vi "Basic.vi"() -> ()   [LabVIEW 2016, in "DronaTest.lvlib" / "test_ValueSignal.lvlib"]
uses:
  test_ValueSignal.lvlib
  main/apis/Setup/GetVI/GetVIByPath.vi
  main/apis/Stimulus/ValueSignal/ValueSignalByPathString.vi
  main/apis/Assert/AssertControlValue/Equal.vi
  main/apis/Assert/AssertControlValue/True.vi
  main/Drona.lvlib
  main/apis/Setup/GetVI/GetVI.lvlib
  <vilib>/addons/_JKI Toolkits/Caraya/classes/Test/Test.lvclass
  main/apis/Stimulus/ValueSignal/ValueSignal.lvlib
  main/apis/Assert/AssertControlValue/AssertControlValue.lvlib
panel:
  out "error out":errorcluster
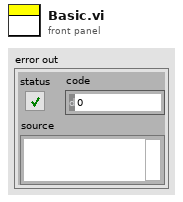
[diagram p1: front panel]
types:
  T1 = cluster{"Numeric_cluster":dbl, "Boolean_cluster":bool, "String_cluster":string}
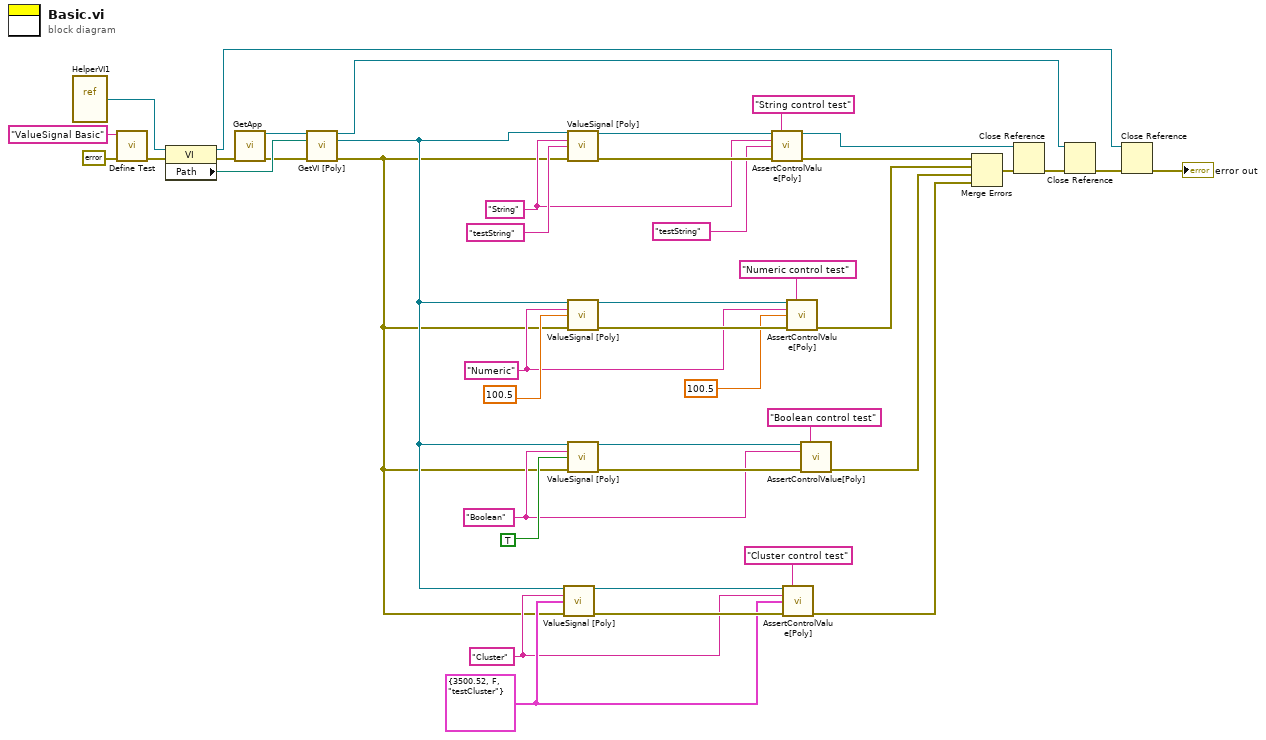
[diagram p0: block diagram]
diagram:
  w3 = "Cluster" ("Control Name")
  w10 = "Boolean" ("Control Name")
  w11 = "Numeric" ("Control Name")
  w12 = "String" ("Control Name")
  w5 = T1 {"Numeric_cluster"=3500.52, "Boolean_cluster"=FALSE, "String_cluster"="testCluster"} ("Cluster")
  n1 = vi-ref "HelperVI1.vi"() -> (w32:refnum<vi>)
  n2 = call <vilib>:"Define Test.vi"("error in (no error)"=errorcluster {"status"=FALSE, "code"=0, "source"=""}, "Label (VI Title)"="ValueSignal Basic") -> ("error out"=w36:errorcluster)  [unwired: 9 in]
  n3 = property on="Property Node" class="VI"(reference=w32, error in=w36) -> (reference out=w34:refnum<vi>, error out=w40:errorcluster, "Path"=w39:path)
  n4 = call "GetApp.vi"("error in (no error)"=w40) -> ("Application Ref"=w41:refnum<vi>, "error out"=w38:errorcluster)  [unwired: 13 in]
  n5 = call-poly "GetVI [Poly].vi"("Application Ref in"=w41, "VI Path"=w39, "error in (no error)"=w38) -> ("Application Ref out"=w33:refnum<vi>, "VI Reference"=w4:refnum<vi>, "error out"=w2:errorcluster)  [unwired: 10 in]
  n6 = call-poly "ValueSignal [Poly].vi"("VI Reference In"=w4, "Control Name"=w3, "Value (Signaling)"=w5, "error in"=w2) -> ("VI Reference Out"=w7:refnum<vi>, "error out"=w6:errorcluster)  [unwired: 10 in]
  n7 = call-poly "ValueSignal [Poly].vi"("VI Reference In"=w4, "Control Name"=w12, "Value (Signaling)"="testString" ("Control Name"), "error in"=w2) -> ("VI Reference Out"=w25:refnum<vi>, "error out"=w27:errorcluster)  [unwired: 10 in]
  n8 = call-poly "ValueSignal [Poly].vi"("VI Reference In"=w4, "Control Name"=w11, "Value (Signaling)"=100.5, "error in"=w2) -> ("VI Reference Out"=w19:refnum<vi>, "error out"=w21:errorcluster)  [unwired: 10 in]
  n9 = call-poly "ValueSignal [Poly].vi"("VI Reference In"=w4, "Control Name"=w10, "Value (Signaling)"=TRUE, "error in"=w2) -> ("VI Reference Out"=w14:refnum<vi>, "error out"=w16:errorcluster)  [unwired: 10 in]
  n10 = call-poly "AssertControlValue[Poly].vi"("VI Reference In"=w25, "Label"="String control test" ("Label (VI Title)"), "Control Name"=w12, "Control Value"="testString" ("Control Name"), "Error In"=w27) -> ("VI Reference Out"=w23:refnum<vi>, "Error Out"=w26:errorcluster)  [unwired: 9 in]
  n11 = call-poly "AssertControlValue[Poly].vi"("VI Reference In"=w7, "Label"="Cluster control test" ("Label (VI Title)"), "Control Name"=w3, "Control Value"=w5, "Error In"=w6) -> ("Error Out"=w1:errorcluster)  [unwired: 9 in, 1 out]
  n12 = call-poly "AssertControlValue[Poly].vi"("VI Reference In"=w19, "Label"="Numeric control test" ("Label (VI Title)"), "Control Name"=w11, "Control Value"=100.5, "Error In"=w21) -> ("Error Out"=w20:errorcluster)  [unwired: 9 in, 1 out]
  n13 = call-poly "AssertControlValue[Poly].vi"("VI Reference In"=w14, "Label"="Boolean control test" ("Label (VI Title)"), "Control Name"=w10, "Error In"=w16) -> ("Error Out"=w15:errorcluster)  [unwired: 10 in, 1 out]
  n14 = Merge Errors(w26, w20, w15, w1) -> (w30:errorcluster)
  n15 = Close Reference(reference=w23, error in (no error)=w30) -> (error out=w9:errorcluster)
  n16 = Close Reference(reference=w33, error in (no error)=w9) -> (error out=w42:errorcluster)
  n17 = Close Reference(reference=w34, error in (no error)=w42) -> (error out=→"error out":errorcluster)
